vi "CG_Auswerten.vi"(7 "Span Auswahl":i32[](array[numeric]), 8 "Istwerte":string[][](array[string]), 9 "Sollwerte":T1[][][](array[typedef]), 10 "Fehler":bool[](array[boolean]), 11 "Zeitstempel":string) -> (2 "Abweichung":string[][](array[string]), 3 "Protokoll":string[](array[string]))   [LabVIEW 2020, in "Erweiterte Konfig.lvlib" / "CG-Check Konfig.lvlib"]
uses:
  CG-Check Konfig.lvlib
  Visualisierungs Elemente/String - Ausgabefeld.ctl
  Aktion_CG-Check.ctl
  CalEingaenge.ctl
  SysLog/SysLog Interface.ctl
  SysLog/SysLog.lvlib
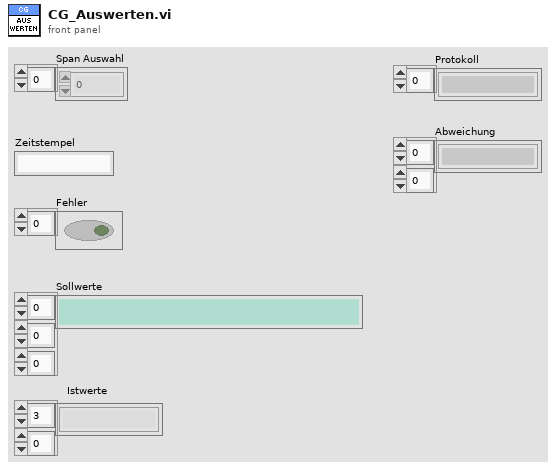
[diagram p1: front panel]
types:
  T1 = typedef "String - Ausgabefeld.ctl" = string
  T2 = typedef "Erweiterte Konfig.lvlib/CG-Check Konfig.lvlib/CalEingaenge.ctl" = string[]
  T3 = typedef "Erweiterte Konfig.lvlib/CG-Check Konfig.lvlib/Aktion_CG-Check.ctl" = enum16{"lesen", "schreiben", "laden", "Komponente", "Aktive?", "speichern"}
  T4 = typedef "SysLog.lvlib/SysLog Interface.ctl" = cluster{"FehlermeldungsCode":i32, "ErfolgsmeldungsCode":i32, "ParameterListenString":string, "Anzeige":bool, "SysLogIcon":enum16{"OK", "Warnung", "Fehler"}, "intern":bool}
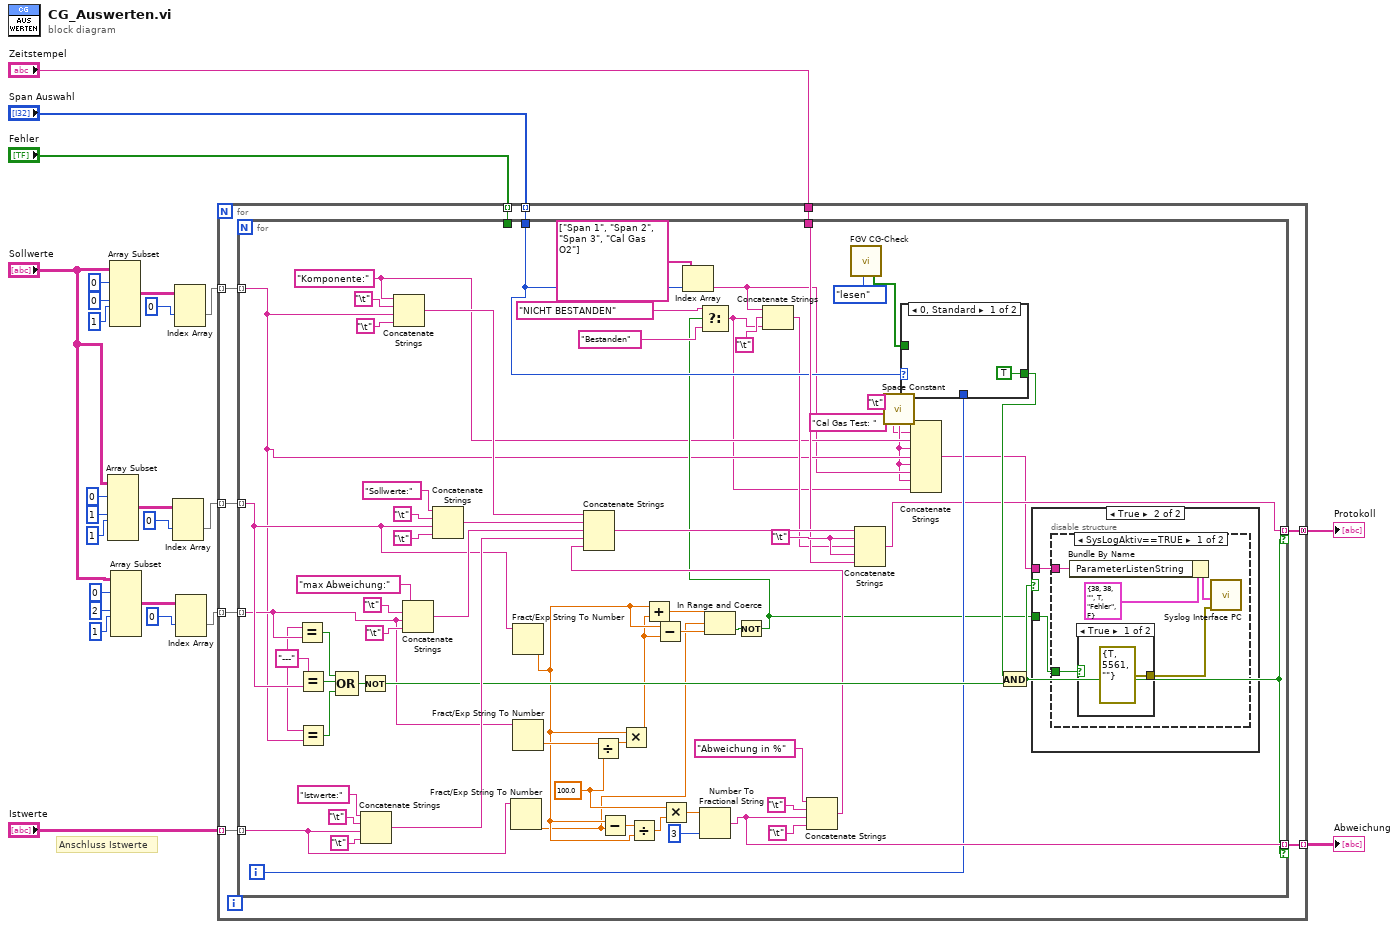
[diagram p0: block diagram]
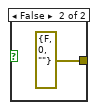
[diagram p3: hidden frame]
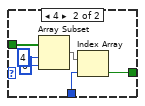
[diagram p5: hidden frame]
diagram:
  # "Anschluss Istwerte"
  n1 = Array Subset(array="Sollwerte", index (dim 0)=0 ("Index"), index (dim 1)=1 ("Index"), length (dim 1)=1 ("Länge")) -> (w10:T1[][][])  [unwired: 3 in]
  n2 = Array Subset(array="Sollwerte", index (dim 0)=0 ("Index"), index (dim 1)=0 ("Index"), length (dim 1)=1 ("Länge")) -> (w7:T1[][][])  [unwired: 3 in]
  n3 = Array Subset(array="Sollwerte", index (dim 0)=0 ("Index"), index (dim 1)=2 ("Index"), length (dim 1)=1 ("Länge")) -> (w18:T1[][][])  [unwired: 3 in]
  n4 = Index Array(array=w10, index (dim 1)=0 ("Index (Seite)")) -> (element=w14:T1[][])  [unwired: 2 in]
  n5 = Index Array(array=w7, index (dim 1)=0 ("Index (Seite)")) -> (element=w6:T1[][])  [unwired: 2 in]
  n6 = Index Array(array=w18, index (dim 1)=0 ("Index (Seite)")) -> (element=w20:T1[][])  [unwired: 2 in]
  n7 = for {
    tunnel: w6 -> [w34] mode=indexing
    tunnel: w14 -> [w33] mode=indexing
    tunnel: w20 -> [w32] mode=indexing
    tunnel: "Istwerte" -> [w31] mode=indexing
    tunnel: [w28] -> w1 mode=concatenating
    tunnel: "Span Auswahl" -> [w30] mode=indexing
    tunnel: "Fehler" -> [w29] mode=indexing
    tunnel: [w27] -> w23 mode=indexing
    tunnel: "Zeitstempel" -> [w26]
    n8 = for {
      tunnel: w34 -> [w39] mode=indexing
      tunnel: w33 -> [w69] mode=indexing
      tunnel: w32 -> [w66] mode=indexing
      tunnel: [w45] -> w28 mode=indexing if=w47
      tunnel: w31 -> [w83] mode=indexing
      tunnel: w30 -> [w48]
      tunnel: w29 -> [_]
      tunnel: [w72] -> w27 mode=indexing if=w47
      tunnel: w26 -> [w67]
      i -> [w52]
      w50 = T1 "---" ("y")
      w64 = 100.0 ("y")
      w68 = "\t"
      w40 = "Komponente:" ("String")
      n9 = Equal?(x=w50, y=w66) -> (x = y?=w97:bool)
      n10 = Equal?(x=w50, y=w69) -> (x = y?=w96:bool)
      n11 = Equal?(x=w50, y=w39) -> (x = y?=w95:bool)
      n12 = Compound Arithmetic op=OR ("Mehrfacharithmetik")(w97, w96, w95) -> (w91:bool)
      n13 = Not(x=w91) -> (.not. x?=w73:bool)
      n14 = Concatenate Strings("Istwerte:" ("String"), "\t", w83, "\t") -> (w84:string)
      n15 = Concatenate Strings(w40, "\t", w39, "\t") -> (w41:string)
      n16 = Concatenate Strings("max Abweichung:" ("String"), "\t", w66, "\t") -> (w90:string)
      n17 = Concatenate Strings("Sollwerte:" ("String"), "\t", w69, "\t") -> (w98:string)
      n18 = Fract/Exp String To Number(string=w83) -> (number=w55:dbl)  [unwired: 3 in, 1 out]
      n19 = Fract/Exp String To Number(string=w69) -> (number=w62:dbl)  [unwired: 3 in, 1 out]
      n20 = Fract/Exp String To Number(string=w66) -> (number=w65:dbl)  [unwired: 3 in, 1 out]
      n21 = Divide(x=w65, y=w64) -> (x/y=w63:dbl)
      n22 = Subtract(x=w55, y=w62) -> (x-y=w56:dbl)
      n23 = Multiply(x=w62, y=w63) -> (x*y=w61:dbl)
      n24 = Divide(x=w56, y=w62) -> (x/y=w89:dbl)
      n25 = Add(x=w62, y=w61) -> (x+y=w60:dbl)
      n26 = Subtract(x=w62, y=w61) -> (x-y=w59:dbl)
      n27 = Multiply(x=w64, y=w89) -> (x*y=w57:dbl)
      n28 = Index Array(array=T2 ["Span 1", "Span 2", "Span 3", "Cal Gas O2"], index=w48) -> (element=w38:string)
      n29 = Number To Fractional String(number=w57, precision (6)=i16 3 ("Genauigkeit (6)")) -> (F-format string=w72:string)  [unwired: 2 in]
      n30 = In Range and Coerce(upper limit=w60, x=w55, lower limit=w59) -> (In Range?=w58:bool)  [unwired: 1 out]
      n31 = Not(x=w58) -> (.not. x?=w46:bool)
      n32 = Select(t="NICHT BESTANDEN", s=w46, f="Bestanden") -> (s? t:f=w36:string)
      n33 = Concatenate Strings(w38, "\t", w36) -> (w44:string)
      n34 = Concatenate Strings("Abweichung in %" ("String"), "\t", w72, "\t") -> (w70:string)
      n35 = Concatenate Strings(w41, w98, w90, w84, w70) -> (w92:string)
      n36 = call "FGV CG-Check.vi"("Aktion"=Aktion_CG-Check."lesen") -> ("Aktive?"=w54:bool[])  [unwired: 11 in, 7 out]
      n37 = Concatenate Strings(w92, w68, w44, w68, w67) -> (w45:string)
      n38 = call <vilib>:"Space Constant.vi"() -> ("String"=w37:string)
      n39 = case shown="0, Standard" w48 {
        tunnel: w54 -> [_ w116]
        tunnel: w52 -> [_ w112]
        tunnel: [TRUE ("Messgas - Eingang 6") w111] -> w51
        frame 0, Default {
        }
        frame 4 {
          n40 = Array Subset(array=w116, index=4 ("Index"), length=6 ("Länge")) -> (w113:bool[])
          n41 = Index Array(array=w113, index=w112) -> (element=w111:bool)
        }
      }
      n42 = Concatenate Strings("Cal Gas Test: " ("String"), "\t", w40, w37, w39, w37, w38, w37, w36) -> (w43:string)
      n43 = And(x=w51, y=w73) -> (x .and. y?=w47:bool)
      n44 = case shown="True" w47 {
        tunnel: w43 -> [_ w102]
        tunnel: w46 -> [_ w101]
        frame False {
        }
        frame True {
          n45 = disable-structure shown="SysLogAktiv==TRUE" {
            disable-tunnel: w102 -> [w103 _]
            disable-tunnel: w101 -> [w106 _]
            frame condition #0 (active) {
              n46 = Bundle By Name(cluster=T4 {"FehlermeldungsCode"=38, "ErfolgsmeldungsCode"=38, "ParameterListenString"="", "Anzeige"=TRUE, "SysLogIcon"=enum."Fehler", "intern"=FALSE} ("Cluster (in)"), "ParameterListenString"=w103) -> (w104:T4)
              n47 = case shown="True" w106 {
                tunnel: [errorcluster {"status"=TRUE, "code"=5561, "source"=""} ("Fehler (in)") errorcluster {"status"=FALSE, "code"=0, "source"=""} ("Fehler (in)")] -> w107
                frame True {
                }
                frame False {
                }
              }
              n48 = call "Syslog Interface PC.vi"("Fehler (in)"=w107, "Cluster (in)"=w104) -> ()  [unwired: 9 in, 1 out]
            }
            frame condition #1 {
            }
          }
        }
      }
    }
  }
  "Abweichung" <- w23
  "Protokoll" <- w1
